vi "plate image.vi"(8 "Slide (mm)":T1={"top"=-22300.0, "right"=-13000.0, "width"=60000.0, "height"=60000.0}, 9 "Y (um)":dbl, 10 "X (um)":dbl, 11 "Stage Limits (mm)":T2={"Y Min"=-4.5, "Y Max"=3.0, "X Min"=-19.0, "X Max"=33.5}) -> (3 "2D Picture":picture)   [LabVIEW 2018]
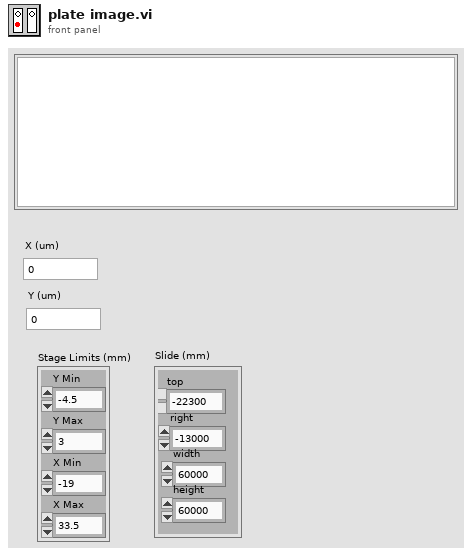
[diagram p1: front panel]
types:
  T1 = cluster{"top":dbl, "right":dbl, "width":dbl, "height":dbl}
  T2 = cluster{"Y Min":dbl, "Y Max":dbl, "X Min":dbl, "X Max":dbl}
  T3 = cluster{"Width":i16, "Style":enum32{"Solid", "Dash", "Dot", "DashDot", "DashDotDot"}}
  T4 = cluster{"left":i16, "top":i16, "right":i16, "bottom":i16}
  T5 = typedef "imagedata.ctl" = cluster{"image type":i32, "image depth":i32, "image":u8[], "mask":u8[], "colors":u32[], "Rectangle":cluster{"left":i16, "top":i16, "right":i16, "bottom":i16}}
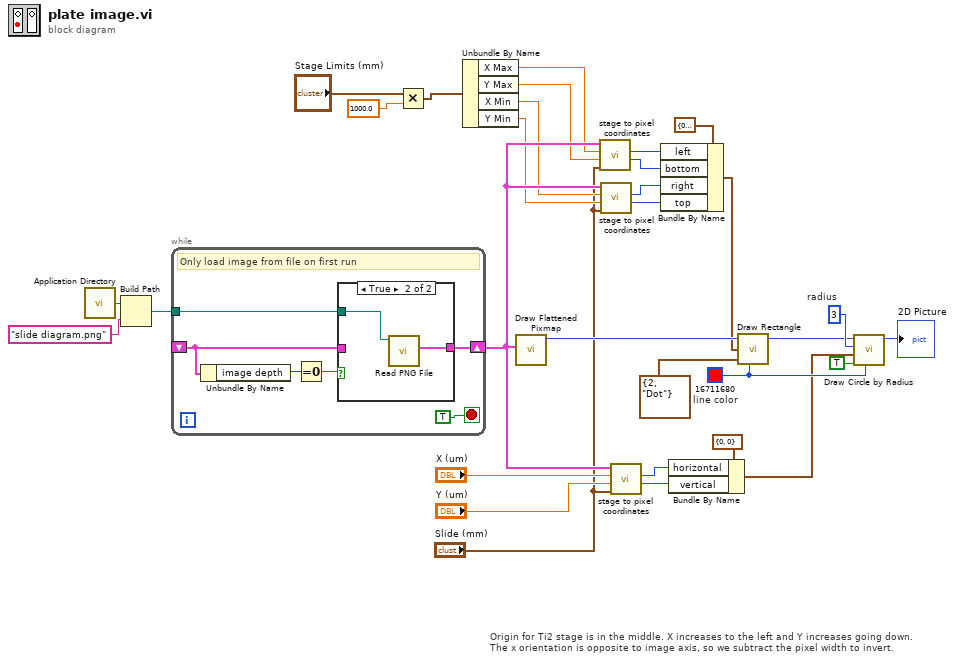
[diagram p0: block diagram]
diagram:
  w31 = i16 3  # radius
  w24 = u32 16711680  # line color
  # "Origin for Ti2 stage is in the middle. X increases to the left and Y increases going down.\nThe x orientation is opposite to image axis, so we subtract the pixel width to invert."
  n1 = call <vilib>:"Application Directory.vi"() -> ("Application Directory"=w1:path)
  n2 = Build Path(base path=w1, name or relative path="slide diagram.png") -> (appended path=w27:path)
  n3 = while {
    tunnel: w27 -> [w36]
    shift-right: [w35] -> w13
    shift-left: _ -> [w33]
    stop <- TRUE stop-if-true
    # "Only load image from file on first run"
    n4 = Unbundle By Name(w33) -> ("image depth"=w34:i32)
    n5 = Equal To 0?(x=w34) -> (x = 0?=w32:bool)
    n6 = case shown="True" w32 {
      tunnel: w36 -> [_ w40]
      tunnel: [w38 w39] -> w35
      tunnel: w33 -> [w38 _]
      frame False {
      }
      frame True {
        n7 = call <vilib>:"Read PNG File.vi"("path to PNG file"=w40) -> ("image data"=w39:T5)  [unwired: 8 in, 2 out]
      }
    }
  }
  n8 = Multiply(x="Stage Limits (mm)", y=1000.0) -> (x*y=w5:T2)
  n9 = Unbundle By Name(w5) -> ("X Max"=w10:dbl, "Y Max"=w9:dbl, "X Min"=w7:dbl, "Y Min"=w8:dbl)
  n10 = call <vilib>:"Draw Flattened Pixmap.vi"("image data"=w13) -> ("new picture"=w26:picture)  [unwired: 8 in]
  n11 = call "stage to pixel coordinates.vi"("Slide (mm)"="Slide (mm)", "Y in (um)"=w9, "X in (um)"=w10, "image data"=w13) -> ("Y out (px)"=w11:i16, "X out (um)"=w12:i16)  [unwired: 6 in]
  n12 = call "stage to pixel coordinates.vi"("Slide (mm)"="Slide (mm)", "Y in (um)"=w8, "X in (um)"=w7, "image data"=w13) -> ("Y out (px)"=w14:i16, "X out (um)"=w15:i16)  [unwired: 6 in]
  n13 = call "stage to pixel coordinates.vi"("Slide (mm)"="Slide (mm)", "Y in (um)"="Y (um)", "X in (um)"="X (um)", "image data"=w13) -> ("Y out (px)"=w19:i16, "X out (um)"=w20:i16)  [unwired: 6 in]
  n14 = Bundle By Name(cluster=T4 {"left"=0, "top"=0, "right"=0, "bottom"=0} ("rect"), "left"=w12, "bottom"=w11, "right"=w15, "top"=w14) -> (w16:T4)
  n15 = Bundle By Name(cluster=cluster{"horizontal":i16, "vertical":i16} {"horizontal"=0, "vertical"=0} ("pixel center"), "horizontal"=w20, "vertical"=w19) -> (w18:cluster{"horizontal":i16, "vertical":i16})
  n16 = call <vilib>:"Draw Rectangle.vi"("picture"=w26, "rect"=w16, "color(black)"=w24, "pen"=T3 {"Width"=2, "Style"=enum."Dot"}) -> ("new picture"=w25:picture)  [unwired: 5 in]
  n17 = call <vilib>:"Draw Circle by Radius.vi"("color(black)"=w24, "fill?(F)"=TRUE, "pixel center"=w18, "radius"=w31, "picture"=w25) -> ("new picture"=→"2D Picture":picture)  [unwired: 6 in]
